vi "TellMediator.vi"(6 "Error":errorcluster, 10 "Message":refnum<class "Message.lvclass">, 11 "Actor":refnum<class "Actor.lvclass">) -> (3 "Actor":refnum<class "Actor.lvclass">, 4 "Error":errorcluster)   [LabVIEW 2020, in "jettl.lvlib"]
uses:
  jettl.lvlib
  TellOriginEnum.ctl
  Actor/Actor.lvclass
  Message/Message.lvclass
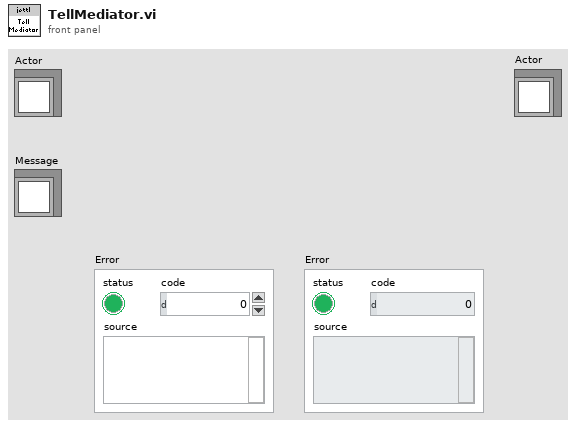
[diagram p1: front panel]
types:
  T1 = typedef "jettl.lvlib/TellOriginEnum.ctl" = enum16{"Self", "Mediator", "Component"}
  T2 = typedef "jettl.lvlib/BaseCluster.ctl" = cluster{"LifecycleEnum":T3, "MainCluster":T4, "SelfActorCluster":T5, "MediatorActorCluster":T5, "ComponentActorClusterMap":T10}
  T3 = typedef "jettl.lvlib/LifecycleEnum.ctl" = enum16{"Initializing", "SettingUp", "Starting", "Running", "Stopping", "TearingDown", "Terminated", "Abort"}
  T4 = typedef "jettl.lvlib/MainCluster.ctl" = cluster{"PreSetupClusterQueue":refnum<queue>, "BeginSetupQueue":refnum<queue>, "PostSetupClusterQueue":refnum<queue>, "BeginStartQueue":refnum<queue>}
  T5 = typedef "jettl.lvlib/ActorCluster.ctl" = cluster{"MessagesCluster":T6, "Alias":string, "ActorTypeEnum":T9, "MessageClusterDVREvent":refnum<user-event>, "EventRegistrationRef":refnum<event-registration>, "VIRef":refnum<vi>}
  T6 = typedef "jettl.lvlib/MessagesCluster.ctl" = cluster{"ListenMessageSet":T7, "TellSelfMessageSet":T7, "TellMediatorMessageSet":T7, "TellComponentMessageSetMap":T8}
  T7 = typedef "jettl.lvlib/MessageSet.ctl" = set{refnum<class "Message.lvclass">}
  T8 = typedef "jettl.lvlib/TellComponentMessageSetMap.ctl" = map{string, T7}
  T9 = typedef "jettl.lvlib/ActorTypeEnum.ctl" = enum16{"Mediator", "Component"}
  T10 = typedef "jettl.lvlib/ComponentActorClusterMap.ctl" = map{string, T5}
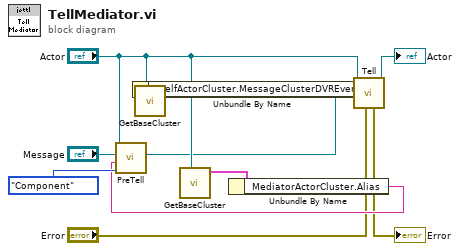
[diagram p0: block diagram]
diagram:
  n1 = call-dynamic "GetBaseCluster.vi"("Actor"="Actor") -> ("BaseCluster"=w9:T2)  [unwired: 10 in]
  n2 = Unbundle By Name(w9) -> ("SelfActorCluster.MessageClusterDVREvent"=w8:refnum<user-event>)
  n3 = call-dynamic "GetBaseCluster.vi"("Actor"="Actor") -> ("BaseCluster"=w5:T2)  [unwired: 10 in]
  n4 = Unbundle By Name(w5) -> ("MediatorActorCluster.Alias"=w4:string)
  n5 = call "PreTell.vi"("TellOriginEnum"=TellOriginEnum."Component" ("TellOrigin"), "ListenerAlias"=w4, "Message"="Message", "Actor"="Actor") -> ("Message"=w3:refnum<class "Message.lvclass">)  [unwired: 7 in]
  n6 = call "Tell.vi"("Error"="Error", "Message"=w3, "MessageClusterDVREvent"=w8, "Actor"="Actor") -> ("Actor"=→"Actor":refnum<class "Actor.lvclass">, "Error"=→"Error":errorcluster)  [unwired: 6 in]
